vi "generate-toolkit-web.vi"() -> ()   [LabVIEW 2010]
uses:
  controls/state-machine.ctl
panel:
  in  "Excluded folders":string[](array[string])=["exportedVis", "exportedVis-old", "PMutil", "PMutil_before_030608", "PMutil-tutu"]
  in  "main index name":string="MTA Applications"
  in  "VIs base path":path=path "/user/pma/PM_app86"
  in  "report file destination":path=path "/doc"
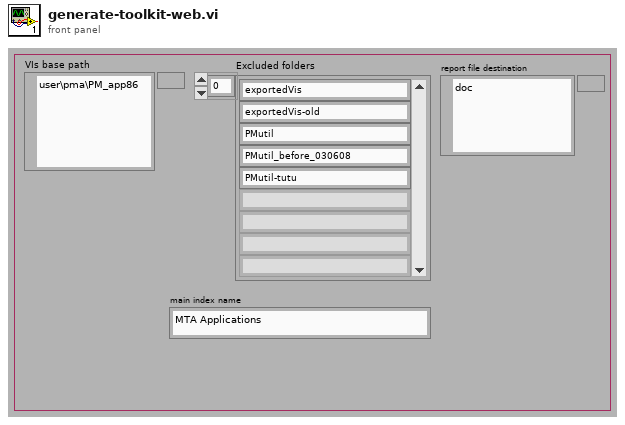
[diagram p1: front panel]
types:
  T1 = typedef "state-machine.ctl" = enum16{"add carridge return", "init", "Read-inputs", "edit generated file", "end", "Add front panel", "Add Block Diagram", "Add VI icon", "Add VI description", "Add VI hiearchy", "Add list of sub vis", "add custom html", "open report in browser", "Save report to file", "dispose report", "Add header text", "Create style .css", "add-red-box-header", "Delete Temp Files", "Remove-path-element", "add-revision-history", "add-icon-image-only"}
  T2 = typedef "state program.ctl" = cluster{"State machine":T1, "HTML before":string, "HTML after":string}
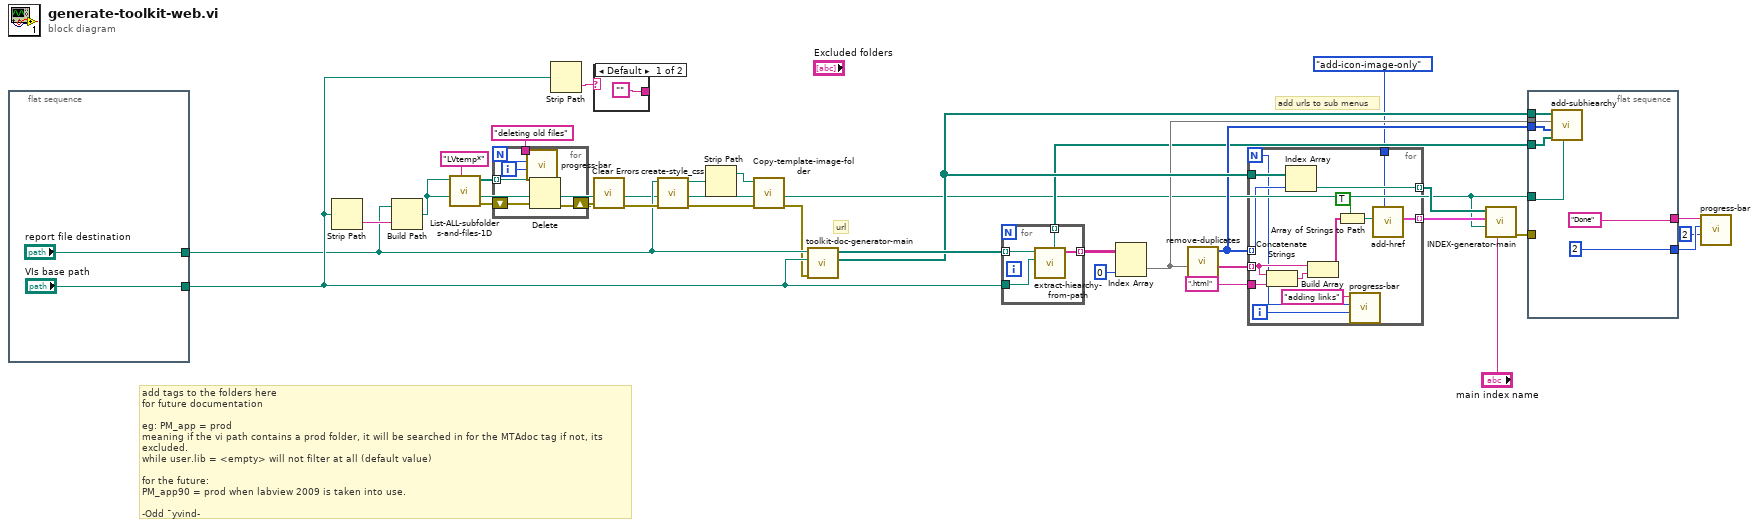
[diagram p0: block diagram]
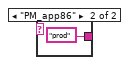
[diagram p2: hidden frame]
diagram:
  # "add tags to the folders here \nfor future documentation\n\neg: PM_app = prod \nmeaning if the vi path contains a prod folder, it will be searched in for the MTAdoc tag if not, its excluded.\nwhile user.lib = <empty> will not filter at all (default value)\n\nfor the future:\nPM_app90 = prod when labview 2009 is taken into use.\n\n-Odd ¯yvind-"
  # "add urls to sub menus"
  # "url"
  n1 = flat-sequence {
    tunnel: ["VIs base path"] -> w11
    tunnel: ["report file destination"] -> w5
    frame #0 {
    }
  }
  n2 = Strip Path(path=w11) -> (name=w26:string)  [unwired: 1 out]
  n3 = Build Path(base path=w5, name or relative path=w26) -> (appended path=w4:path)
  n4 = call "List-ALL-subfolders-and-files-1D.vi"("pattern"="LVtemp*", "Top level folder"=w4) -> ("error IO"=w18:errorcluster, "files found"=w19:path[])  [unwired: 1 in, 7 out]
  n5 = for {
    N -> [w37]
    tunnel: w19 -> [w40] mode=indexing
    shift-right: [w38] -> w17
    shift-left: w18 -> [w39]
    tunnel: "deleting old files" ("state") -> [w35]
    i -> [w36]
    n6 = call "progress-bar.vi"("i++"=w36, "max"=w37, "state"=w35) -> ()  [unwired: 9 out]
    n7 = Delete(path (use dialog)=w40, error in=w39) -> (error out=w38:errorcluster)  [unwired: 5 out]
  }
  n8 = Strip Path(path=w11) -> (name=w10:string)  [unwired: 1 out]
  n9 = case shown="Default" w10 {
    tunnel: ["" "prod"] -> _
    frame Default {
    }
    frame "PM_app86" {
    }
  }
  n10 = call <vilib>:"Clear Errors.vi"("error in (no error)"=w17) -> ("error out"=w7:errorcluster)  [unwired: 6 out]
  n11 = call "create-style_css.vi"("error in (no error)"=w7, "path to .css file"=w5) -> ("error out"=w6:errorcluster, "path"=w9:path)  [unwired: 8 out]
  n12 = Strip Path(path=w9) -> (stripped path=w8:path)  [unwired: 1 out]
  n13 = call "Copy-template-image-folder.vi"("error in"=w6, "target path (use dialog)"=w8) -> ("error out"=w3:errorcluster)  [unwired: 9 out]
  n14 = call "toolkit-doc-generator-main.vi"("error in"=w3, "VIs base path"=w11, "report file destination"=w5) -> ("vi paths"=w25:path[], "htmls generated"=w32:path[])  [unwired: 3 in, 4 out]
  n15 = for {
    tunnel: w11 -> [w46]
    tunnel: w32 -> [w45] mode=indexing
    tunnel: [w44] -> w31 mode=indexing
    tunnel: [w43] -> w22 mode=indexing
    n16 = call "extract-hiearchy-from-path.vi"("base"=w46, "location"=w45) -> ("Array"=w44:string[], "relative path"=w43:path)  [unwired: 8 out]
  }
  n17 = Index Array(array=w31, index (col)=0 ("disabled index (col)")) -> (element=w24:string[])  [unwired: 1 in]
  n18 = call "remove-duplicates.vi"("Input Array"=w24) -> ("Output Array"=w29:string[], "indices of kept elements"=w23:i32[])  [unwired: 1 in, 8 out]
  n19 = for {
    N -> [w50]
    tunnel: w23 -> [w59] mode=indexing
    tunnel: w25 -> [w60]
    tunnel: [w58] -> w27 mode=indexing
    tunnel: [w57] -> w28 mode=indexing
    tunnel: w29 -> [w51] mode=indexing
    tunnel: ".html" ("string") -> [w54]
    tunnel: state-machine."add-icon-image-only" ("State machine") -> [w47]
    i -> [w49]
    n20 = Concatenate Strings(w51, w54) -> (w53:string)
    n21 = Index Array(array=w60, index=w59) -> (element=w58:path)
    n22 = Build Array(w51, w53) -> (w52:string[])
    n23 = Array of Strings to Path(0:w52, 1:TRUE ("relative")) -> (2:w56:path)
    n24 = call "progress-bar.vi"("i++"=w49, "max"=w50, "state"="adding links") -> ()  [unwired: 9 out]
    n25 = call "add-href.vi"("State machine"=w47, "relative path"=w56) -> ("state"=w57:T2)  [unwired: 9 out]
  }
  n26 = call "INDEX-generator-main.vi"("header"="main index name", "report file destination"=w4, "tasks"=w28, "VI paths"=w27) -> ("error out"=w16:errorcluster)  [unwired: 2 in, 5 out]
  n27 = flat-sequence {
    tunnel: w25 -> [w67]
    tunnel: w24 -> [w66]
    tunnel: w23 -> [w65]
    tunnel: w22 -> [w64]
    tunnel: w4 -> [w61]
    tunnel: w16 -> [_]
    tunnel: ["Done"] -> w14
    tunnel: [2 ("max")] -> w13
    frame #0 {
      n28 = call "add-subhiearchy.vi"("appended path"=w61, "all relative paths"=w64, "indices of kept elements"=w65, "tree main structure"=w66, "all vi paths"=w67) -> ()  [unwired: 7 out]
    }
  }
  n29 = call "progress-bar.vi"("i++"=u32 2, "max"=w13, "state"=w14) -> ()  [unwired: 9 out]
